vi "WS1050 CV Register Cntrl.vi"(8 "error in (no error)":errorcluster, 10 "CV Reg Setting":i32(ring)=1 items=["All OFF", "Reg 1 ON", "Reg 2 ON", "Reg 3 ON", "All ON"], 11 "Com Port":refnum<visa-resource-name>) -> (0 "error out":errorcluster, 3 "Com Port Out":refnum<visa-resource-name>)   [LabVIEW 2012]
panel:
  out "number":i32
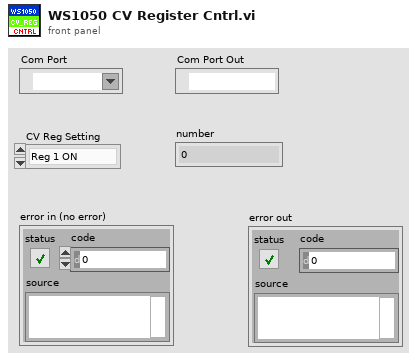
[diagram p1: front panel]
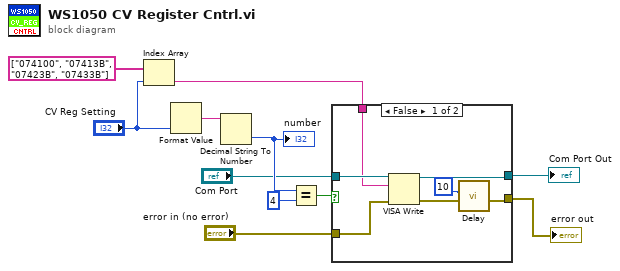
[diagram p0: block diagram]
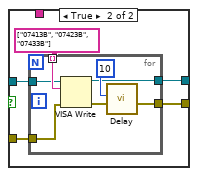
[diagram p2: hidden frame]
diagram:
  n1 = Index Array(array=string[] ["074100", "07413B", "07423B", "07433B"], index="CV Reg Setting") -> (element=w3:string)
  n2 = Format Value(value (0)="CV Reg Setting") -> (output string=w9:string)  [unwired: 2 in]
  n3 = Decimal String To Number(string=w9) -> (number=w7:i32)  [unwired: 2 in, 1 out]
  "number" <- w7
  n4 = Equal?(x=w7, y=4) -> (x = y?=w8:bool)
  n5 = case shown="False" w8 {
    tunnel: [w18 w22] -> w4
    tunnel: "Com Port" -> [w13 w21]
    tunnel: w3 -> [w12 _]
    tunnel: "error in (no error)" -> [w14 w20]
    tunnel: [w16 w19] -> w1
    frame False {
      n6 = VISA Write(VISA resource name=w13, write buffer=w12, error in (no error)=w14) -> (VISA resource name out=w18:refnum<visa-resource-name>, error out=w15:errorcluster)  [unwired: 1 out]
      n7 = call "Delay.vi"("error in (no error)"=w15, "milliseconds to wait"=u32 10) -> ("error out"=w16:errorcluster)  [unwired: 9 in]
    }
    frame True {
      n8 = for {
        tunnel: string[] ["07413B", "07423B", "07433B"] -> [w28] mode=indexing
        tunnel: [w27] -> w22
        tunnel: w21 -> [w26]
        tunnel: w20 -> [w25]
        tunnel: [w24] -> w19
        n9 = VISA Write(VISA resource name=w26, write buffer=w28, error in (no error)=w25) -> (VISA resource name out=w27:refnum<visa-resource-name>, error out=w30:errorcluster)  [unwired: 1 out]
        n10 = call "Delay.vi"("error in (no error)"=w30, "milliseconds to wait"=u32 10) -> ("error out"=w24:errorcluster)  [unwired: 9 in]
      }
    }
  }
  "Com Port Out" <- w4
  "error out" <- w1
